vi "Format File Property.vi"(8 "Error In":errorcluster, 9 "File Property Value":string, 10 "File Property Name":string, 11 "String in":string) -> (0 "Error Out":errorcluster, 3 "String out":string)   [LabVIEW 2024]
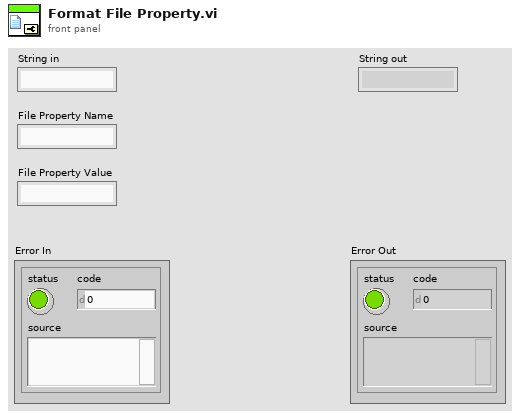
[diagram p1: front panel]
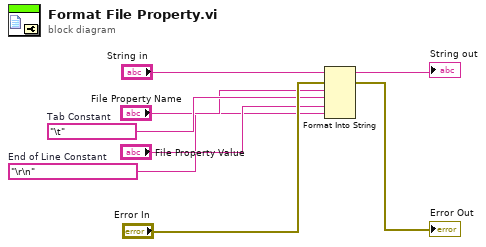
[diagram p0: block diagram]
diagram:
  w3 = "\r\n"  # End of Line Constant
  w6 = "\t"  # Tab Constant
  n1 = Format Into String(initial string="String in", error in="Error In", "File Property Name", w6, "File Property Value", w3) -> (resulting string=→"String out":string, error out=→"Error Out":errorcluster)  [unwired: 1 in]
